vi "CheckReferenceValue.vi"(10 "YCoordIn":sgl format="%#_13g", 11 "XCoordIn":sgl format="%#_13g") -> (2 "YCoordOut":sgl format="%#_13g", 3 "XCoordOut":sgl format="%#_13g")   [LabVIEW 2017]
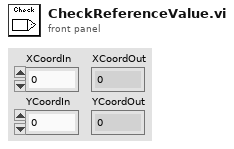
[diagram p1: front panel]
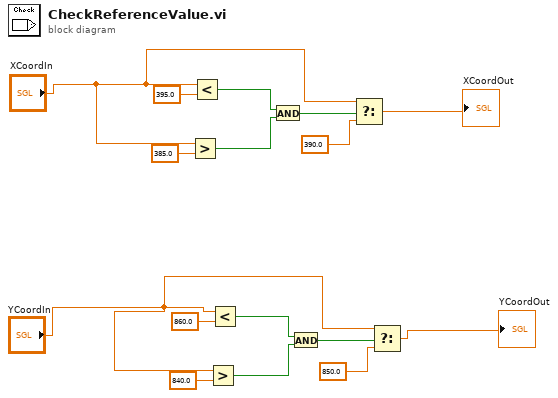
[diagram p0: block diagram]
diagram:
  n1 = Greater?(x="XCoordIn", y=sgl 385.0) -> (0:w15:bool)
  n2 = Less?(x="XCoordIn", y=sgl 395.0) -> (x < y?=w16:bool)
  n3 = Greater?(x="YCoordIn", y=sgl 840.0) -> (0:w7:bool)
  n4 = Less?(x="YCoordIn", y=sgl 860.0) -> (x < y?=w8:bool)
  n5 = And(x=w16, y=w15) -> (x .and. y?=w10:bool)
  n6 = And(x=w8, y=w7) -> (x .and. y?=w3:bool)
  n7 = Select(t="XCoordIn", s=w10, f=sgl 390.0 ("y")) -> (s? t:f=→"XCoordOut":sgl)
  n8 = Select(t="YCoordIn", s=w3, f=sgl 850.0 ("y")) -> (s? t:f=→"YCoordOut":sgl)
